vi "Write First_.vi"(8 "error in (no error)":errorcluster, 10 "First?":bool, 11 "BCAdmin in":refnum<class "BCAdmin.lvclass">) -> (0 "error out":errorcluster, 3 "BCAdmin out":refnum<class "BCAdmin.lvclass">)   [LabVIEW 2014, in "BusController.lvlib" / "BCAdmin.lvclass"]
uses:
  BCAdmin.lvclass
  BCAdmin.lvclass/BCAdmin.ctl
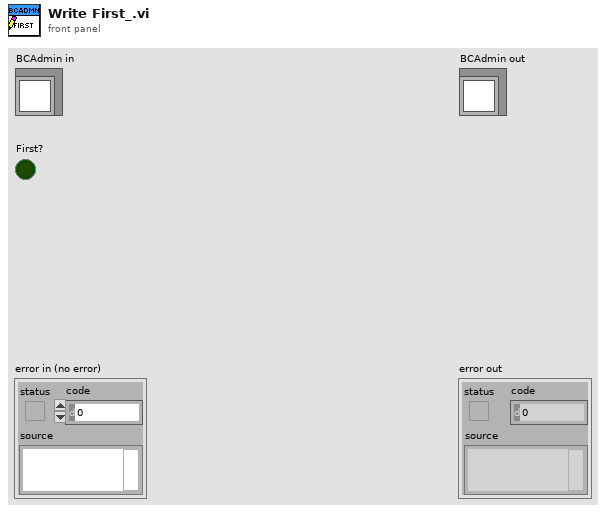
[diagram p1: front panel]
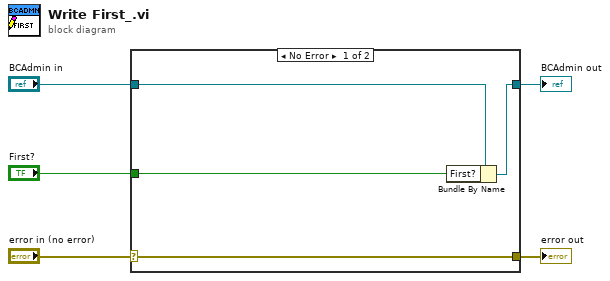
[diagram p0: block diagram]
diagram:
  n1 = case shown="No Error" "error in (no error)" {
    selector: "error in (no error)" -> [w9 w10]
    tunnel: [w9 w10] -> w4
    tunnel: [w7 w11] -> w2
    tunnel: "BCAdmin in" -> [w8 w11]
    tunnel: "First?" -> [w6 _]
    frame No Error {
      n2 = Bundle By Name(cluster=w8, "First?"=w6) -> (w7:refnum<class "BCAdmin.lvclass">)
    }
    frame Error {
    }
  }
  "error out" <- w4
  "BCAdmin out" <- w2
